vi "Extract from Start and End Timestamps.vi"(8 "Error":errorcluster, 9 "Stop Out":timestamp format="%<%M:%S%u.2>T", 10 "Start Out":timestamp format="%<%M:%S%u.2>T", 11 "(WavBuf)":refnum<class "(WavBuf).lvclass">) -> (0 "Error Out":errorcluster, 1 "Start Out":i32, 2 "Buffer Out":T1, 3 "(WavBuf) Out":refnum<class "(WavBuf).lvclass">, 4 "End Out":i32)   [LabVIEW 2016, in "(WavBuf).lvclass"]
uses:
  (WavBuf).lvclass
  Universal Controls/Waveform_Data.ctl
  (WavBuf).lvclass/(WavBuf).ctl
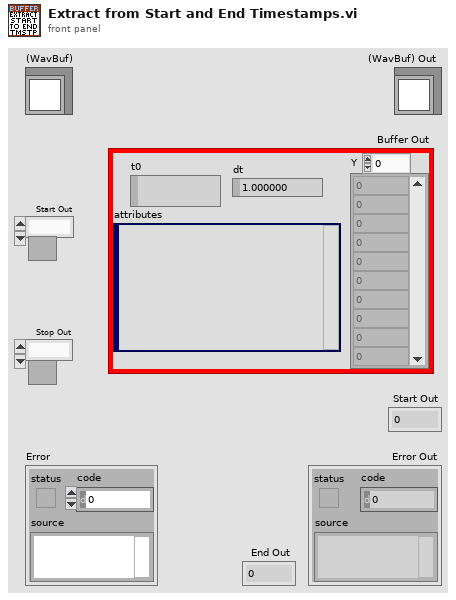
[diagram p1: front panel]
types:
  T1 = typedef "Waveform_Data.ctl" = waveform(dbl)
  T2 = typedef "Ref_DVR_Buffer.ctl" = refnum<data-value>
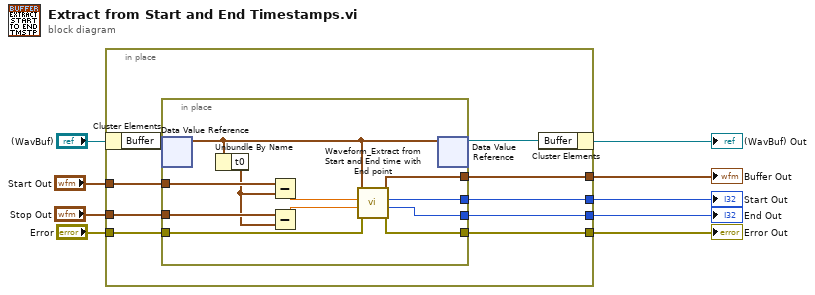
[diagram p0: block diagram]
diagram:
  n1 = in-place {
    in-place-border: "Error" -> [w18]
    in-place-border: [w17] -> w5
    in-place-border: [w16] -> w3
    in-place-border: [w15] -> w8
    in-place-border: [w14] -> w7
    in-place-border: "Start Out" -> [w13]
    in-place-border: "Stop Out" -> [w12]
    n2 = in-place-cluster #1("(WavBuf)") -> ("Buffer"=w11:T2)
    n3 = in-place {
      in-place-border: w18 -> [w29]
      in-place-border: [w28] -> w17
      in-place-border: [w25] -> w16
      in-place-border: [w26] -> w15
      in-place-border: [w27] -> w14
      in-place-border: w13 -> [w23]
      in-place-border: w12 -> [w22]
      n4 = in-place-dvr #2(w11) -> (w24:T1)  [unwired: 1 out]
      n5 = Unbundle By Name(w24) -> ("t0"=w21:timestamp)
      n6 = Subtract(x=w23, y=w21) -> (x-y=w20:dbl)
      n7 = Subtract(x=w22, y=w21) -> (x-y=w19:dbl)
      n8 = call "Waveform_Extract from Start and End time with End point.vi"("Error"=w29, "End Time"=w19, "Begin Time"=w20, "Waveform"=w24) -> ("Error Out"=w28:errorcluster, "End Index Out"=w27:i32, "Start Index Out"=w26:i32, "Waveform Out"=w25:T1)  [unwired: 4 in]
      n9 = in-place-dvr #2(w24) -> (w10:T2)  [unwired: 1 out]
    }
    n10 = in-place-cluster #1("Buffer"=w10) -> (→"(WavBuf) Out":refnum<class "(WavBuf).lvclass">)
  }
  "Error Out" <- w5
  "Buffer Out" <- w3
  "Start Out" <- w8
  "End Out" <- w7
